vi "LJM_OpenS.vi"(8 "error in":errorcluster, 9 "Identifier":string="LJM_idANY", 10 "ConnectionType":string="LJM_ctANY", 11 "DeviceType":string="LJM_dtANY") -> (0 "error out":errorcluster, 3 "Handle":i32)   [LabVIEW 2019]
uses:
  labjackm.dll
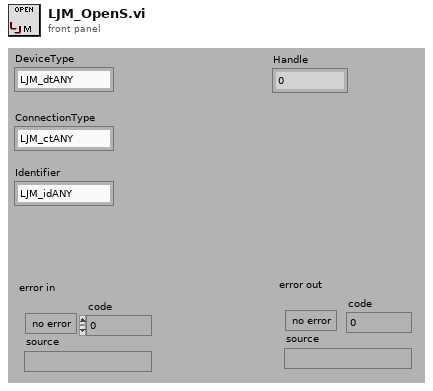
[diagram p1: front panel]
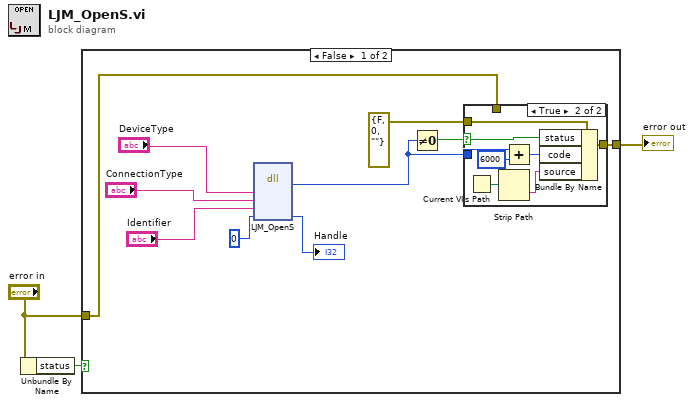
[diagram p0: block diagram]
diagram:
  n1 = Unbundle By Name("error in") -> ("status"=w2:bool)
  n2 = case shown="False" w2 {
    tunnel: [w9 w23] -> w3
    tunnel: "error in" -> [w8 w23]
    frame False {
      n3 = dll-call lib="labjackm.dll" fn="LJM_OpenS"("DeviceType"="DeviceType", "ConnectionType"="ConnectionType", "Identifier"="Identifier", "Handle"=0) -> (w10:i32, "Handle"=→"Handle":i32)  [unwired: 6 in, 2 out]
      n4 = Not Equal To 0?(x=w10) -> (x != 0?=w11:bool)
      n5 = case shown="True" w11 {
        selector: w11 -> [_ w21]
        tunnel: [w14 w22] -> w9
        tunnel: errorcluster {"status"=FALSE, "code"=0, "source"=""} ("error IO") -> [_ w20]
        tunnel: w10 -> [_ w16]
        tunnel: w8 -> [w14 _]
        frame False {
        }
        frame True {
          n6 = Current VI's Path() -> (path=w18:path)
          n7 = Strip Path(path=w18) -> (name=w19:string)  [unwired: 1 out]
          n8 = Add(x=w16, y=6000) -> (x+y=w17:i32)
          n9 = Bundle By Name(cluster=w20, "status"=w21, "code"=w17, "source"=w19) -> (w22:errorcluster)
        }
      }
    }
    frame True {
    }
  }
  "error out" <- w3
